vi "servo movement.vi"   [LabVIEW 2010, in "Tank Robot.lvrbt"]
uses:
  Tank Robot.lvrbt
  <vilib>/NXT/Subs/LVHSConnector.ctl
  <vilib>/NXT/NXTIO Xnodes/AddressXNode/NXTIOAddress.xnode
  <vilib>/NXT/Subs/MotorXNode.Servo Type.ctl
  <vilib>/NXT/Subs/MotorXNode.1Servo.ctl
  <vilib>/NXT/NXTIO Xnodes/NXTIOXNode/NXTIO.xnode
  <vilib>/NXT/NXTIO Xnodes/NXTIONodeSubVIs/TETRIX IO Move Servos.vi
  <vilib>/NXT/Dual Mode Library/Display/drawNumber_float.vi
types:
  T1 = typedef "MotorXNode.Servo Type.ctl" = enum16{"Servo"}
  T2 = typedef "FTC ControllerState.ctl" = cluster{"Left X":i8, "Left Y":i8, "Right X":i8, "Right Y":i8, "Button Encoding 9-12":u8, "Button Encoding 1-8":u8, "POV":T3}
  T3 = typedef "FTC POVState.ctl" = i8
  T4 = typedef "FTC ButtonState.ctl" = cluster{"Button 1":bool, "Button 2":bool, "Button 3":bool, "Button 4":bool, "Button 5":bool, "Button 6":bool, "Button 7":bool, "Button 8":bool, "Button 9":bool, "Button 10":bool, "Button 11":bool, "Button 12":bool, "POV":T3}
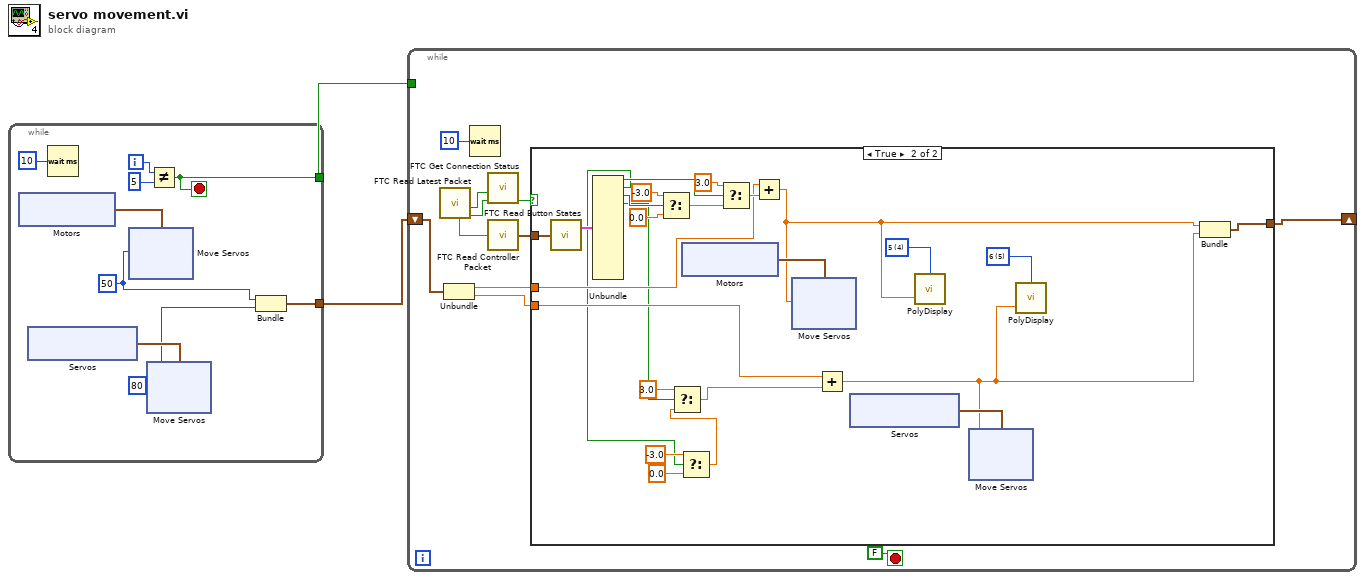
[diagram p0: block diagram]
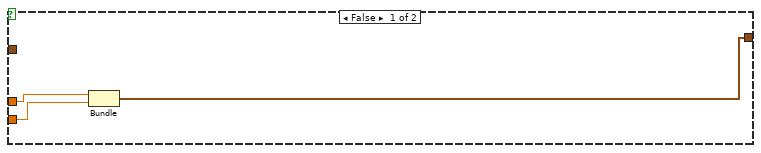
[diagram p2: hidden frame]
diagram:
  n1 = while {
    tunnel: [w7] -> w2
    tunnel: [w3] -> w1
    i -> [w11]
    stop <- w7 stop-if-true
    w4 = u8 80 ("Position 1")
    w5 = u8 50 ("Position 1")
    n2 = xnode "Motors"() -> ("Servo"=w8:cluster{"Servo":T1, "Address":i16})
    n3 = xnode "Servos"() -> ("Servo"=w6:cluster{"Servo":T1, "Address":i16})
    n4 = Wait (ms)(milliseconds to wait=u32 10) -> ()  [unwired: 1 out]
    n5 = xnode "Move Servos"("Position 1"=w5, "Servos"=w8) -> ()  [unwired: 1 in, 1 out]
    n6 = xnode "Move Servos"("Position 1"=w4, "Servos"=w6) -> ()  [unwired: 1 in, 1 out]
    n7 = Not Equal?(x=w11, y=5) -> (x != y?=w7:bool)
    n8 = Bundle("Position 1"=w5, "Position 1"=w4) -> (w3:cluster{"Position 1":u8, "Position 1":u8})  [unwired: 1 in]
  }
  n9 = while {
    tunnel: w2 -> [_]
    shift-right: [w33] -> _
    shift-left: w1 -> [w32]
    stop <- FALSE stop-if-true
    n10 = call <vilib>:"FTC Read Latest Packet.vi"() -> ("Packet Received?"=w37:bool, "Stopped?"=w38:bool, "Controller 1"=w35:string)  [unwired: 6 in, 3 out]
    n11 = Unbundle(w32) -> ("Position 1"=w31:dbl, "Position 1"=w30:dbl)
    n12 = Wait (ms)(milliseconds to wait=u32 10) -> ()  [unwired: 1 out]
    n13 = call <vilib>:"FTC Get Connection Status.vi"("Packet Received?"=w37, "Stopped?"=w38) -> ("Online?"=w36:bool)  [unwired: 6 in, 2 out]
    n14 = call <vilib>:"FTC Read Controller Packet.vi"("Packet"=w35) -> ("Controller State"=w34:T2)  [unwired: 4 in]
    n15 = case shown="True" w36 {
      tunnel: w34 -> [_ w68]
      tunnel: [w41 w53] -> w33
      tunnel: w31 -> [w43 w52]
      tunnel: w30 -> [w42 w51]
      frame False {
        n16 = Bundle("Position 1"=w43, "Position 1"=w42) -> (w41:cluster{"Position 1":dbl, "Position 1":dbl})  [unwired: 1 in]
      }
      frame True {
        w44 = i16 5 items=["1", "2", "3", "4", "5", "6", "7", "8"] ("Line")
        w46 = i16 4 items=["1", "2", "3", "4", "5", "6", "7", "8"] ("Line")
        n17 = call <vilib>:"FTC Read Button States.vi"("Controller State"=w68) -> ("Button States"=w67:T4)  [unwired: 2 in, 1 out]
        n18 = Unbundle(w67) -> ("Button 1"=w66:bool, "Button 2"=w48:bool, "Button 3"=w61:bool, "Button 4"=w49:bool)  [unwired: 9 out]
        n19 = Select(t=-3.0, s=w61, f=0.0) -> (s? t:f=w64:dbl)
        n20 = Select(t=-3.0, s=w48, f=0.0) -> (s? t:f=w58:dbl)
        n21 = Select(t=3.0, s=w49, f=w58) -> (s? t:f=w54:dbl)
        n22 = xnode "Motors"() -> ("Servo"=w59:cluster{"Servo":T1, "Address":i16})
        n23 = Select(t=3.0, s=w66, f=w64) -> (s? t:f=w60:dbl)
        n24 = Add(x=w52, y=w60) -> (x+y=w47:dbl)
        n25 = xnode "Move Servos"("Position 1"=w47, "Servos"=w59) -> ()  [unwired: 1 in, 1 out]
        n26 = Add(x=w51, y=w54) -> (x+y=w45:dbl)
        n27 = xnode "Servos"() -> ("Servo"=w50:cluster{"Servo":T1, "Address":i16})
        n28 = call-poly <vilib>:"PolyDisplay.vi"("number"=w47, "Line"=w46) -> ()  [unwired: 2 in, 1 out]
        n29 = xnode "Move Servos"("Position 1"=w45, "Servos"=w50) -> ()  [unwired: 1 in, 1 out]
        n30 = call-poly <vilib>:"PolyDisplay.vi"("number"=w45, "Line"=w44) -> ()  [unwired: 2 in, 1 out]
        n31 = Bundle(w47, w45) -> (w53:cluster{dbl, dbl})  [unwired: 1 in]
      }
    }
  }
